vi "Validate if event is selected.vi"(11 "Tree Selection":string) -> (0 "Selection type":T1=enum."Broadcast")   [LabVIEW 2019, in "Panther Dashboard.lvlib"]
uses:
  Panther Dashboard.lvlib
  Selection Type--enum.ctl
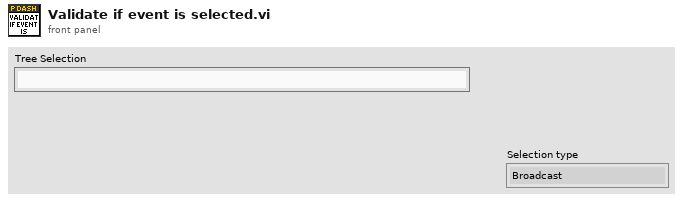
[diagram p1: front panel]
types:
  T1 = typedef "Panther Dashboard.lvlib/Selection Type--enum.ctl" = enum16{"Module", "Public API", "Broadcast", "Request", "Request and Wait for Reply"}
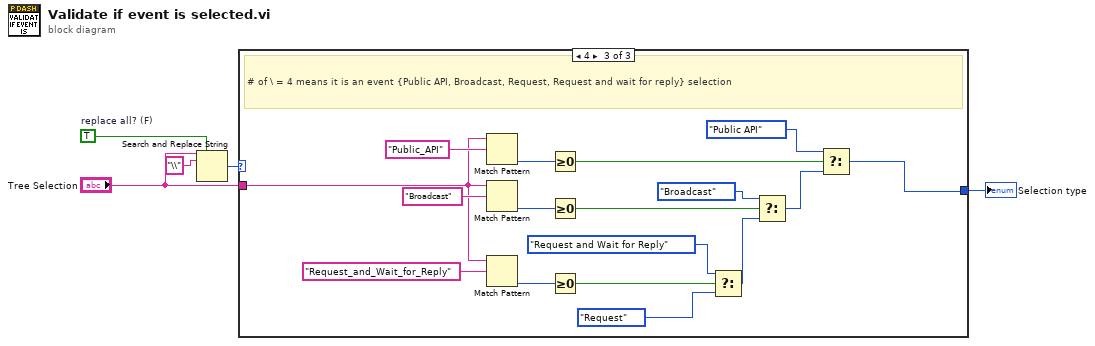
[diagram p0: block diagram]
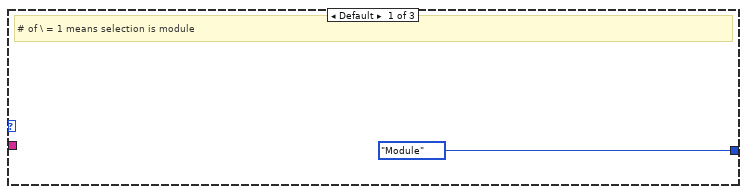
[diagram p2: hidden frame]
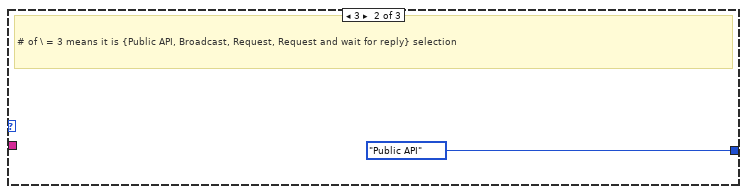
[diagram p3: hidden frame]
diagram:
  w4 = TRUE  # replace all? (F)
  n1 = Search and Replace String(replace all?=w4, input string="Tree Selection", search string="\\") -> (number of replacements=w3:i32)  [unwired: 5 in, 3 out]
  n2 = case shown="4" w3 {
    tunnel: [Selection_Type--enum."Module" Selection_Type--enum."Public API" w20] -> w1
    tunnel: "Tree Selection" -> [_ _ w14]
    frame Default {
      # "# of \\ = 1 means selection is module"
    }
    frame 3 {
      # "# of \\ = 3 means it is {Public API, Broadcast, Request, Request and wait for reply} selection"
    }
    frame 4 {
      # "# of \\ = 4 means it is an event {Public API, Broadcast, Request, Request and wait for reply} selection"
      n3 = Match Pattern(string=w14, regular expression="Public_API") -> (offset past match=w23:i32)  [unwired: 1 in, 3 out]
      n4 = Match Pattern(string=w14, regular expression="Broadcast") -> (offset past match=w18:i32)  [unwired: 1 in, 3 out]
      n5 = Match Pattern(string=w14, regular expression="Request_and_Wait_for_Reply") -> (offset past match=w12:i32)  [unwired: 1 in, 3 out]
      n6 = Greater Or Equal To 0?(x=w23) -> (x >= 0?=w22:bool)
      n7 = Greater Or Equal To 0?(x=w18) -> (x >= 0?=w17:bool)
      n8 = Greater Or Equal To 0?(x=w12) -> (x >= 0?=w11:bool)
      n9 = Select(t=Selection_Type--enum."Request and Wait for Reply", s=w11, f=Selection_Type--enum."Request") -> (s? t:f=w9:T1)
      n10 = Select(t=Selection_Type--enum."Broadcast", s=w17, f=w9) -> (s? t:f=w15:T1)
      n11 = Select(t=Selection_Type--enum."Public API", s=w22, f=w15) -> (s? t:f=w20:T1)
    }
  }
  "Selection type" <- w1
